vi "Fix path [array].vi"(8 "error in (no error)":errorcluster, 10 "Paths in":string[](array[string]), 11 "File Transfer Behavior in":refnum<class "File Transfer Behavior.lvclass">) -> (0 "error out":errorcluster, 2 "Paths out":string[](array[string]), 3 "File Transfer Behavior out":refnum<class "File Transfer Behavior.lvclass">)   [LabVIEW 2015, in "RT Management.lvlib" / "File Transfer Behavior.lvclass"]
doc: "The path is correctly configured to work in as many situations as possible. Any given path should be returned by this VI in the form \"/path1/path2/path3\", where path1 does not equal \"C\", \"C:\", \"c\", or \"c:\".\n\nFor example, the path \"C:\\blah\\directory\\\" would be transformed to \"/blah/directory\".\n\nThe path in may not contain the characters \"\\\" or \"/\" in their filename. Otherwise, this VI may return an invalid path and/or the path was invalid to begin with."
uses:
  File Transfer Behavior.lvclass
  <vilib>/Utility/error.llb/Trim Whitespace.vi
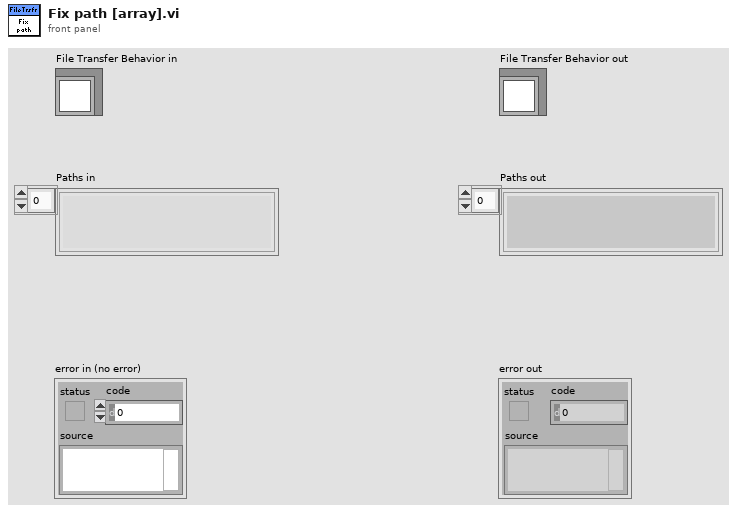
[diagram p1: front panel]
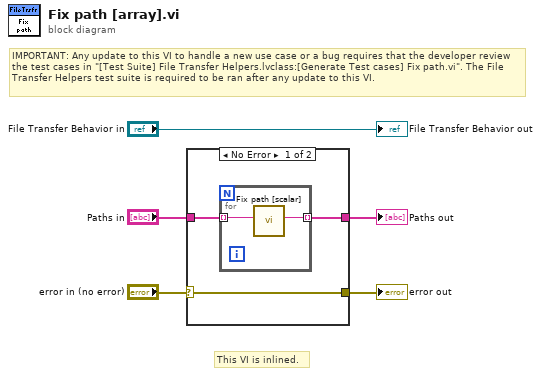
[diagram p0: block diagram]
diagram:
  # "This VI is inlined."
  # "IMPORTANT: Any update to this VI to handle a new use case or a bug requires that the developer review the test cases in \"[Test Suite] File Transfer Helpers.lvclass:[Generate Test cases] Fix path.vi\". The File Transfer Helpers test suite is required to be ran after any update to this VI."
  n1 = case shown="No Error" "error in (no error)" {
    selector: "error in (no error)" -> [w6 w12]
    tunnel: [w6 w12] -> w4
    tunnel: "Paths in" -> [w8 w11]
    tunnel: [w7 w11] -> w2
    frame No Error {
      n2 = for {
        tunnel: w8 -> [w9] mode=indexing
        tunnel: [w10] -> w7 mode=indexing
        n3 = call "Fix path [scalar].vi"("Path in"=w9) -> ("Path out"=w10:string)  [unwired: 8 in, 2 out]
      }
    }
    frame Error {
    }
  }
  "error out" <- w4
  "Paths out" <- w2
  "File Transfer Behavior out" <- "File Transfer Behavior in"
